vi "SLL DE AO Command LV2Global.vi"(6 "Option":T2=enum."Get Event Refnum", 8 "Error in (no error)":errorcluster, 10 "Execute For":string, 11 "AO Option":T1) -> (0 "Error out":errorcluster, 3 "Event Registration Refnum":refnum<event-registration>)   [LabVIEW 2013]
uses:
  Controls/SLL DE AO Command LV2Global Options.ctl
  Controls/SLL DE AO Global Options.ctl
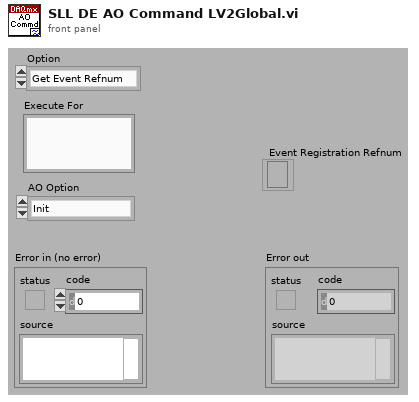
[diagram p1: front panel]
types:
  T1 = typedef "SLL DE AO Global Options.ctl" = enum16{"Init", "Write Line", "Write Array", "Read Line", "Read Array", "Read Full Status", "Restart AO", "Send to Safe Mode", "Stop AO"}
  T2 = typedef "SLL DE AO Command LV2Global Options.ctl" = enum16{"Init/Register Events", "Get Event Refnum", "Fire Event", "Distroy Event"}
  T3 = cluster{"User Event":refnum<user-event>, "Event Registration Refnum":refnum<event-registration>}
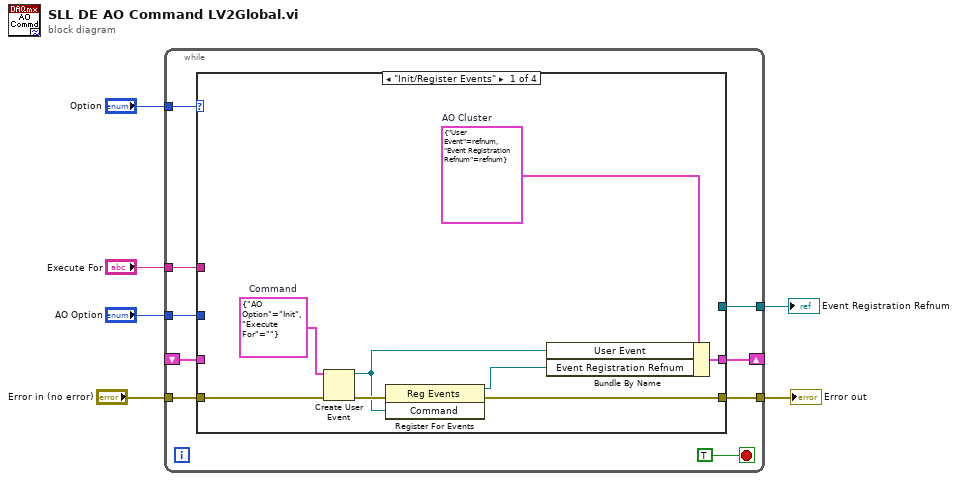
[diagram p0: block diagram]
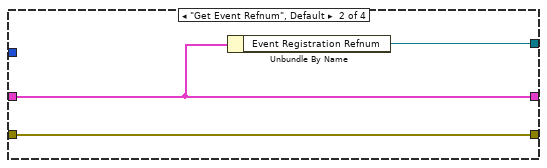
[diagram p2: hidden frame]
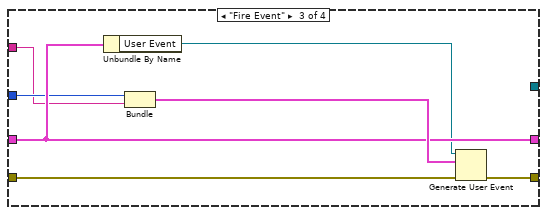
[diagram p3: hidden frame]
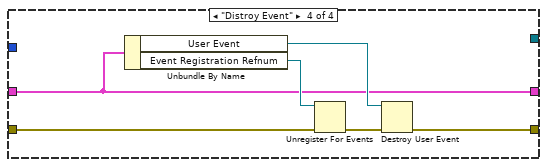
[diagram p4: hidden frame]
diagram:
  n1 = while {
    tunnel: "Option" -> [w14]
    shift-right: [w13] -> _
    shift-left: _ -> [w12]
    tunnel: "AO Option" -> [w11]
    tunnel: [w10] -> w4
    tunnel: "Error in (no error)" -> [w9]
    tunnel: [w8] -> w2
    tunnel: "Execute For" -> [w7]
    stop <- TRUE stop-if-true
    n2 = case shown="\"Init/Register Events\"" w14 {
      tunnel: [w20 w25 w32 w34] -> w13
      tunnel: w12 -> [_ w25 w32 w34]
      tunnel: w11 -> [_ _ w28 _]
      tunnel: [w19 w26 w29 w35] -> w10
      tunnel: w9 -> [w18 w26 w30 w36]
      tunnel: [_ w24 _ _] -> w8
      tunnel: w7 -> [_ _ w27 _]
      frame "Init/Register Events" {
        w23 = T3 {"User Event"=refnum, "Event Registration Refnum"=refnum}  # AO Cluster
        w21 = cluster{"AO Option":T1, "Execute For":string} {"AO Option"=enum."Init", "Execute For"=""}  # Command
        n3 = Create User Event(user event datatype=w21, error in=w18) -> (user event=w17:refnum<user-event>, error out=w22:errorcluster)
        n4 = register-events(error in=w22, w17) -> (reference out=w16:refnum<event-registration>, error out=w19:errorcluster)  [unwired: 1 in]
        n5 = Bundle By Name(cluster=w23, "User Event"=w17, "Event Registration Refnum"=w16) -> (w20:T3)
      }
      frame "Get Event Refnum", Default {
        n6 = Unbundle By Name(w25) -> ("Event Registration Refnum"=w24:refnum<event-registration>)
      }
      frame "Fire Event" {
        n7 = Unbundle By Name(w32) -> ("User Event"=w31:refnum<user-event>)
        n8 = Bundle("AO Option"=w28, "Execute For"=w27) -> (w33:cluster{"AO Option":T1, "Execute For":string})  [unwired: 1 in]
        n9 = Generate User Event(user event=w31, event data cluster=w33, error in=w30) -> (error out=w29:errorcluster)  [unwired: 1 in, 1 out]
      }
      frame "Distroy Event" {
        n10 = Unbundle By Name(w34) -> ("User Event"=w39:refnum<user-event>, "Event Registration Refnum"=w37:refnum<event-registration>)
        n11 = Unregister For Events(event registration refnum=w37, error in=w36) -> (error out=w38:errorcluster)
        n12 = Destroy User Event(user event=w39, error in=w38) -> (error out=w35:errorcluster)
      }
    }
  }
  "Error out" <- w4
  "Event Registration Refnum" <- w2
